vi "FTW-TestExecutive-Sequence-Interpret.vi"(0 "JSON":string, 11 "error in":errorcluster) -> (4 "Sequence":T1[](array[typedef]) {"Results"."Start Time" format="%<%Y-%m-%d %H:%M:%S%03u>T"; "Results"."Elapsed Time" format="%<%H:%M:%S%3u>t"; "Elapsed Time" format="%<%H:%M:%S%3u>t"}, 15 "error out":errorcluster)   [LabVIEW 2018]
doc: "Can be used to interpret the following messages\n\nSequenceLoaded\nSequenceComplete\nStepChange"
uses:
  FTW-TestExecutive-Step.ctl
  FTW-TestExecutive-Step-State.ctl
  FTW-TestExecutive-Results.ctl
  fe25cb45-b961-4e43-8b8d-ea049e2cfd06.vi
  JSON/core/FTW-JSON-Core-EncodingFlags.vi
  Reflection/FTW-Reflection-Type.vi
  JSON/FTW-JSON-Parse.vi
  container/FTW-Container-GetFlattenedValue.vi
  container/FTW-Container.lvclass
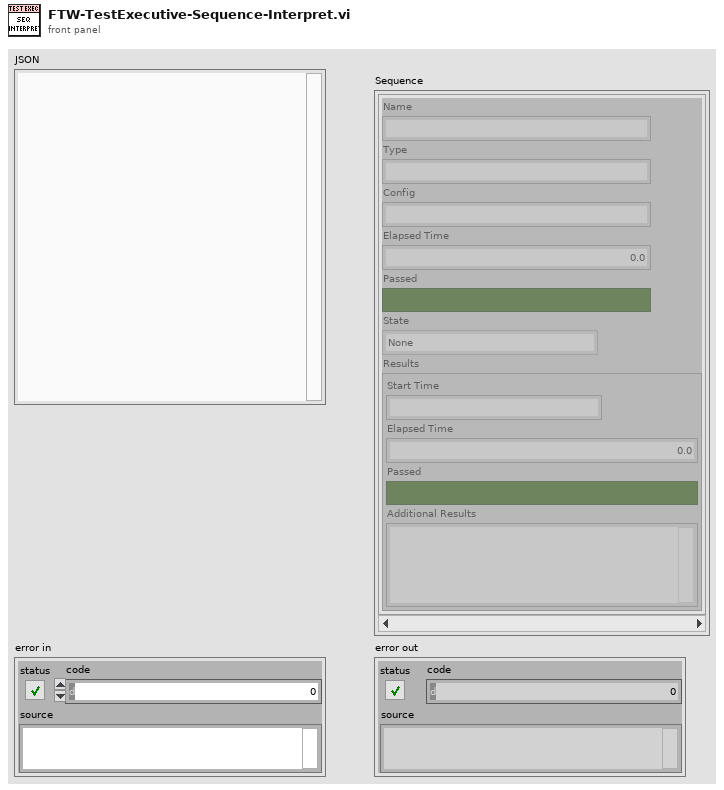
[diagram p1: front panel]
types:
  T1 = typedef "FTW-TestExecutive-Step.ctl" = cluster{"Name":string, "Type":string, "Config":string, "Elapsed Time":dbl, "Passed":bool, "State":T2, "Results":T3}
  T2 = typedef "FTW-TestExecutive-Step-State.ctl" = enum8{"None", "Failed", "Passed", "Timed out", "Aborted"}
  T3 = typedef "FTW-TestExecutive-Results.ctl" = cluster{"Start Time":timestamp, "Elapsed Time":dbl, "Passed":bool, "Additional Results":string}
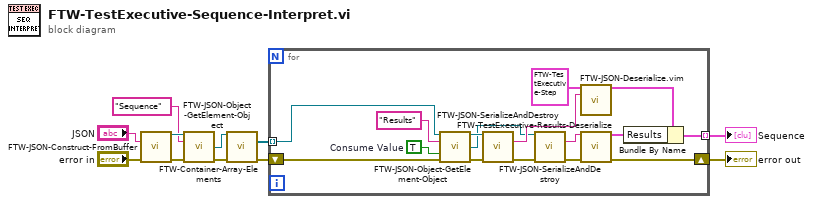
[diagram p0: block diagram]
diagram:
  n1 = call "FTW-JSON-Construct-FromBuffer.vi"("JSON String (UTF-8)"="JSON", "error in"="error in") -> ("JSON"=w7:refnum<class "FTW-Container.lvclass">, "error out"=w9:errorcluster)  [unwired: 12 in]
  n2 = call "FTW-JSON-Object-GetElement-Object.vi"("JSON"=w7, "Key"="Sequence", "error in"=w9) -> ("Value"=w4:refnum<class "FTW-Container.lvclass">, "error out"=w8:errorcluster)  [unwired: 8 in, 3 out]
  n3 = call "FTW-Container-Array-Elements.vi"("FTW-Container In"=w4, "error in"=w8) -> ("Array Elements"=w2:refnum<class "FTW-Container.lvclass">[], "error out"=w5:errorcluster)  [unwired: 11 in, 1 out]
  n4 = for {
    tunnel: w2 -> [w21] mode=indexing
    shift-right: [w25] -> w3
    shift-left: w5 -> [w27]
    tunnel: [w18] -> w1 mode=indexing
    w16 = TRUE  # Consume Value
    n5 = call "FTW-JSON-Object-GetElement-Object.vi"("JSON"=w21, "Key"="Results", "Consume Value"=w16, "error in"=w27) -> ("JSON out"=w20:refnum<class "FTW-Container.lvclass">, "Value"=w14:refnum<class "FTW-Container.lvclass">, "error out"=w22:errorcluster)  [unwired: 7 in, 2 out]
    n6 = call "FTW-JSON-SerializeAndDestroy.vi"("JSON"=w20, "error in"=w22) -> ("JSON String (UTF-8)"=w23:string, "error out"=w26:errorcluster)  [unwired: 12 in]
    n7 = call "FTW-JSON-SerializeAndDestroy.vi"("JSON"=w14, "error in"=w26) -> ("JSON String (UTF-8)"=w13:string, "error out"=w15:errorcluster)  [unwired: 12 in]
    n8 = call "FTW-JSON-Deserialize.vim"("Type In"=T1 {"Name"="", "Type"="", "Config"="", "Elapsed Time"=0.0, "Passed"=FALSE, "State"=enum."None", "Results"={"Start Time"=timestamp(0 s since 1904-01-01), "Elapsed Time"=0.0, "Passed"=FALSE, "Additional Results"=""}} ("Step"), "JSON String"=w23) -> ("Type Out"=w19:T1)  [unwired: 12 in, 1 out]
    n9 = call "FTW-TestExecutive-Results-Deserialize.vi"("Serialized Results"=w13, "error in (no error)"=w15) -> ("Results"=w12:T3, "error out"=w25:errorcluster)  [unwired: 12 in]
    n10 = Bundle By Name(cluster=w19, "Results"=w12) -> (w18:T1)
  }
  "error out" <- w3
  "Sequence" <- w1
